vi "Positions.vi"() -> ()   [LabVIEW 2016]
panel:
  in  "Positions":i32[](array[numeric])
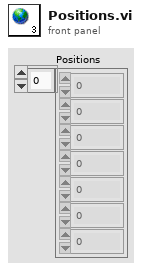
[diagram p1: front panel]
diagram:
